vi "Read Results from processing.vi"(8 "error in":errorcluster, 11 "RT Resource Usage runtime in":refnum<class "RT Resource Usage runtime.lvclass">) -> (0 "error out":errorcluster, 2 "Results from processing":T1, 3 "RT Resource Usage runtime out":refnum<class "RT Resource Usage runtime.lvclass">)   [LabVIEW 2017, in "RT Resource Usage runtime.lvclass"]
uses:
  RT Resource Usage runtime.lvclass
  configuration/result data indices.ctl
  RT Resource Usage runtime.lvclass/RT Resource Usage runtime.ctl
  configuration/RT Resource Usage configuration.lvclass
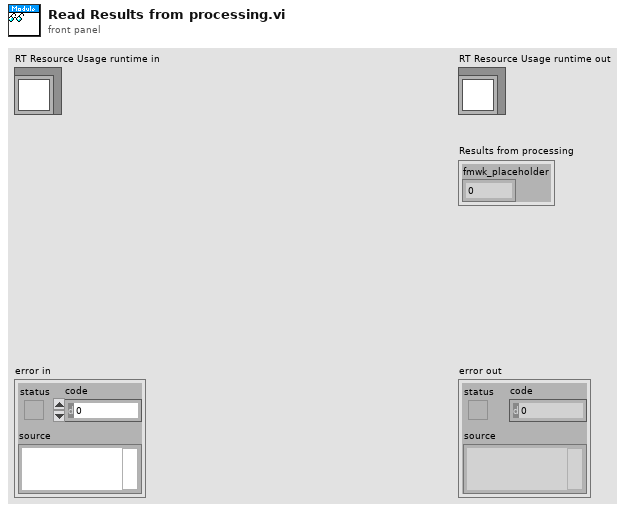
[diagram p1: front panel]
types:
  T1 = typedef "RT Resource Usage configuration.lvclass/result data indices.ctl" = cluster{"fmwk_placeholder":i32}
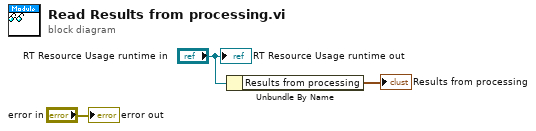
[diagram p0: block diagram]
diagram:
  n1 = Unbundle By Name("RT Resource Usage runtime in") -> ("Results from processing"=→"Results from processing":T1)
  "error out" <- "error in"
  "RT Resource Usage runtime out" <- "RT Resource Usage runtime in"
